vi "DiscArchiver.ProcPeriodic.vi"(0 "i ref in":refnum<vi>, 3 "ms timeout (10000)":i32=10000, 5 "error in (no error)":errorcluster) -> (14 "i ref out":refnum<vi>, 17 "timed out":bool, 19 "error out":errorcluster)   [LabVIEW 2014, in "DiscArchiver.lvlib"]
doc: "This method serves to periodically do things like reading values from the HW. Methods that should be executed periodically should be called from THIS method. Add code here."
uses:
  DiscArchiver.lvlib
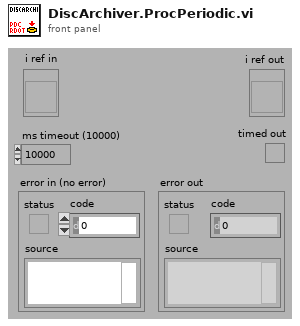
[diagram p1: front panel]
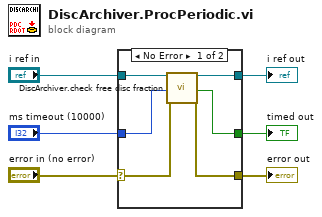
[diagram p0: block diagram]
diagram:
  n1 = case shown="No Error" "error in (no error)" {
    selector: "error in (no error)" -> [w7 w13]
    tunnel: "i ref in" -> [w12 w14]
    tunnel: "ms timeout (10000)" -> [w11 _]
    tunnel: [w10 w14] -> w4
    tunnel: [w9 w13] -> w3
    tunnel: [w8 _] -> w2
    frame No Error {
      n2 = call "DiscArchiver.check free disc fraction.vi"("i ref in"=w12, "ms timeout (10000)"=w11, "error in (no error)"=w7) -> ("i ref out"=w10:refnum<vi>, "timed out"=w8:bool, "error out"=w9:errorcluster)  [unwired: 13 in, 1 out]
    }
    frame Error {
    }
  }
  "error out" <- w3
  "i ref out" <- w4
  "timed out" <- w2
